vi "Nine Leds Off.vi"() -> (3 "LEDs":bool[](array[boolean]))   [LabVIEW 2016]
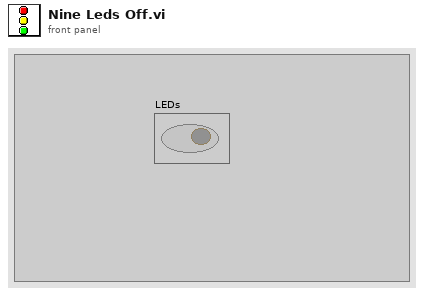
[diagram p1: front panel]
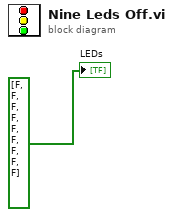
[diagram p0: block diagram]
diagram:
  "LEDs" <- bool[] [FALSE, FALSE, FALSE, FALSE, FALSE, FALSE, FALSE, FALSE, FALSE] ("LEDs")
